vi "Note Result.vi"(8 "error in (no error)":errorcluster, 9 "Stage":enum16{"Init", "Work"}(ring), 10 "Acquired Result.lvclass":refnum<class "Acquired Result.lvclass">, 11 "Response Synchronizer in":refnum<class "Response Synchronizer.lvclass">) -> (0 "error out":errorcluster, 1 "Results":refnum<class "Acquired Result.lvclass">[](array[class]), 2 "Awaiting results":bool, 3 "Response Synchronizer out":refnum<class "Response Synchronizer.lvclass">)   [LabVIEW 2021, in "Response Synchronizer.lvclass"]
uses:
  Response Synchronizer.lvclass
  NHMFL_Core/Libraries/Instruments/Results/Acquired Result/Acquired Result.lvclass
  NHMFL_Core/Libraries/Instruments/Results/Acquired Result/Acquired Result.lvclass/Acquired Result.ctl
  Response Synchronizer.lvclass/Response Synchronizer.ctl
  NHMFL_Core/Libraries/Instruments/Results/Acquired Result/Read Sender.vi
  NHMFL_Core/Libraries/Instruments/Results/Acquired Result/Read Final.vi
  NHMFL_Core/Libraries/Instruments/Results/Acquired Result/Read Cycle count.vi
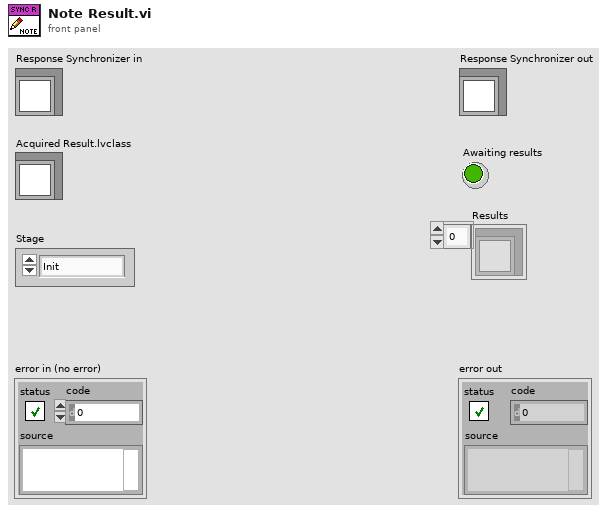
[diagram p1: front panel]
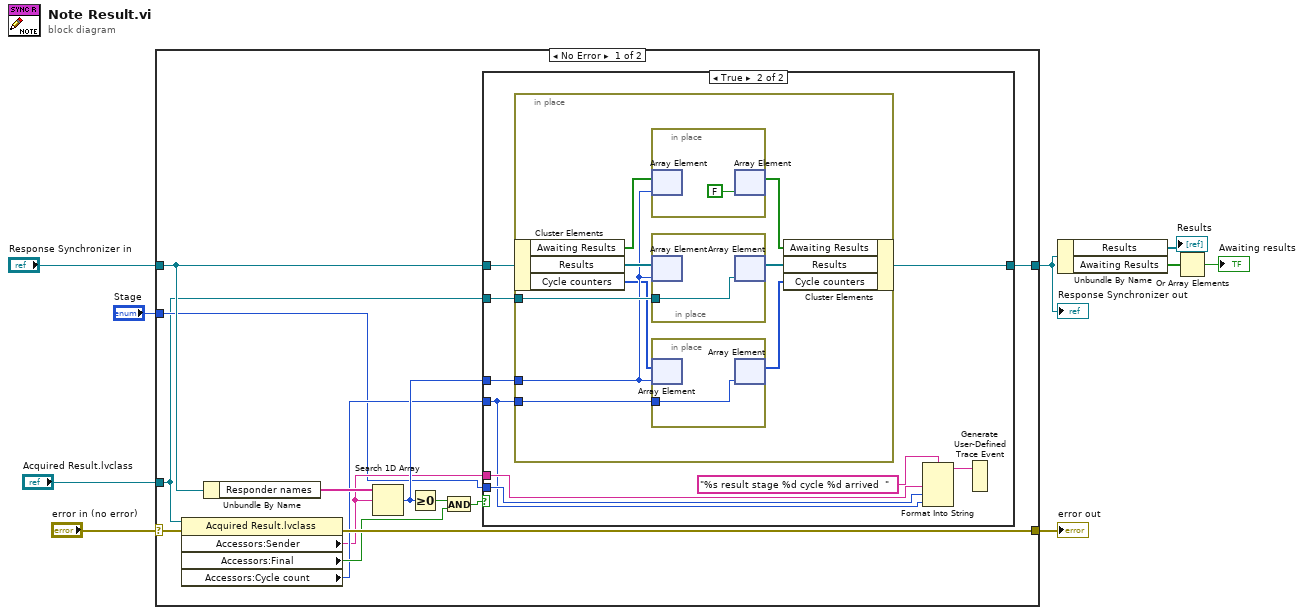
[diagram p0: block diagram]
diagram:
  n1 = case shown="No Error" "error in (no error)" {
    selector: "error in (no error)" -> [w21 w46]
    tunnel: [w20 w46] -> w8
    tunnel: [w18 w45] -> w5
    tunnel: "Response Synchronizer in" -> [w19 w45]
    tunnel: "Stage" -> [w11 _]
    tunnel: "Acquired Result.lvclass" -> [w10 _]
    frame No Error {
      n2 = property class="Acquired Result.lvclass"(reference=w10, error in=w21) -> (error out=w20:errorcluster, "Accessors:Sender"=w12:string, "Accessors:Final"=w14:bool, "Accessors:Cycle count"=w13:i32)  [unwired: 1 out]
      n3 = Unbundle By Name(w19) -> ("Responder names"=w22:string[])
      n4 = Search 1D Array(1D array=w22, element=w12) -> (index of element=w16:i32)  [unwired: 1 in]
      n5 = Greater Or Equal To 0?(x=w16) -> (x >= 0?=w17:bool)
      n6 = And(x=w17, y=w14) -> (x .and. y?=w15:bool)
      n7 = case shown="True" w15 {
        tunnel: w16 -> [_ w32]
        tunnel: w10 -> [_ w31]
        tunnel: w19 -> [w23 w30]
        tunnel: [w23 w29] -> w18
        tunnel: w13 -> [_ w25]
        tunnel: w12 -> [_ w27]
        tunnel: w11 -> [_ w26]
        frame False {
        }
        frame True {
          n8 = in-place {
            in-place-border: w32 -> [w37]
            in-place-border: w31 -> [w39]
            in-place-border: w25 -> [w36]
            n9 = in-place-cluster #1(w30) -> ("Awaiting Results"=w41:bool[], "Results"=w40:refnum<class "Acquired Result.lvclass">[], "Cycle counters"=w35:i32[])
            n10 = in-place {
              n11 = in-place-array #2(w41, w37) -> ()  [unwired: 1 out]
              n12 = in-place-array #2(FALSE ("new element/subarray")) -> (w33:bool[])  [unwired: 1 out]
            }
            n13 = in-place {
              in-place-border: w39 -> [w43]
              n14 = in-place-array #3(w40, w37) -> ()  [unwired: 1 out]
              n15 = in-place-array #3(w43) -> (w38:refnum<class "Acquired Result.lvclass">[])  [unwired: 1 out]
            }
            n16 = in-place {
              in-place-border: w36 -> [w42]
              n17 = in-place-array #4(w35, w37) -> ()  [unwired: 1 out]
              n18 = in-place-array #4(w42) -> (w34:i32[])  [unwired: 1 out]
            }
            n19 = in-place-cluster #1("Awaiting Results"=w33, "Results"=w38, "Cycle counters"=w34) -> (w29:refnum<class "Response Synchronizer.lvclass">)
          }
          n20 = Format Into String(format string="%s result stage %d cycle %d arrived  ", w27, w26, w25) -> (resulting string=w24:string)  [unwired: 2 in, 1 out]
          n21 = Generate User-Defined Trace Event(2:w24) -> ()  [unwired: 1 in]
        }
      }
    }
    frame Error {
    }
  }
  "error out" <- w8
  "Response Synchronizer out" <- w5
  n22 = Unbundle By Name(w5) -> ("Results"=→"Results":refnum<class "Acquired Result.lvclass">[], "Awaiting Results"=w3:bool[])
  n23 = Or Array Elements(Boolean array=w3) -> (logical OR=→"Awaiting results":bool)
